vi "test Get All TPDO Communication Parameter.vi"(11 "Test Case In":refnum<class "Test PDO Mapping.lvclass">) -> (0 "error out":errorcluster, 3 "Test Case Out":refnum<class "Test PDO Mapping.lvclass">)   [LabVIEW 2020, in "Test PDO Mapping.lvclass"]
uses:
  Test PDO Mapping.lvclass
  C:/Program Files/National Instruments/LabVIEW 2026/vi.lib/Astemes/LUnit/Test Case.lvclass
  EDS-File-Viewer/source/Electronic Datasheet/Electronic Datasheet.lvclass/Electronic Datasheet.ctl
  <vilib>/Astemes/LUnit/Test Case.lvclass/Test Case.ctl
  source/PDO Communication Parameter/PDO Communication Parameter.lvclass
  4993e8ee-a06a-463a-9684-69129f64d5ce.vi
  EDS-File-Viewer/source/Electronic Datasheet/Electronic Datasheet.lvclass
  source/CANopen.lvlib
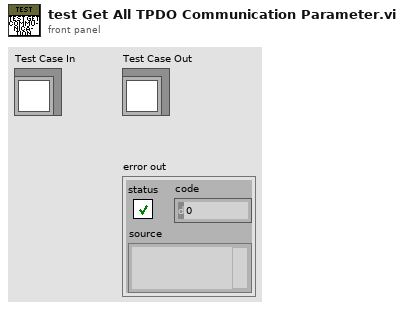
[diagram p1: front panel]
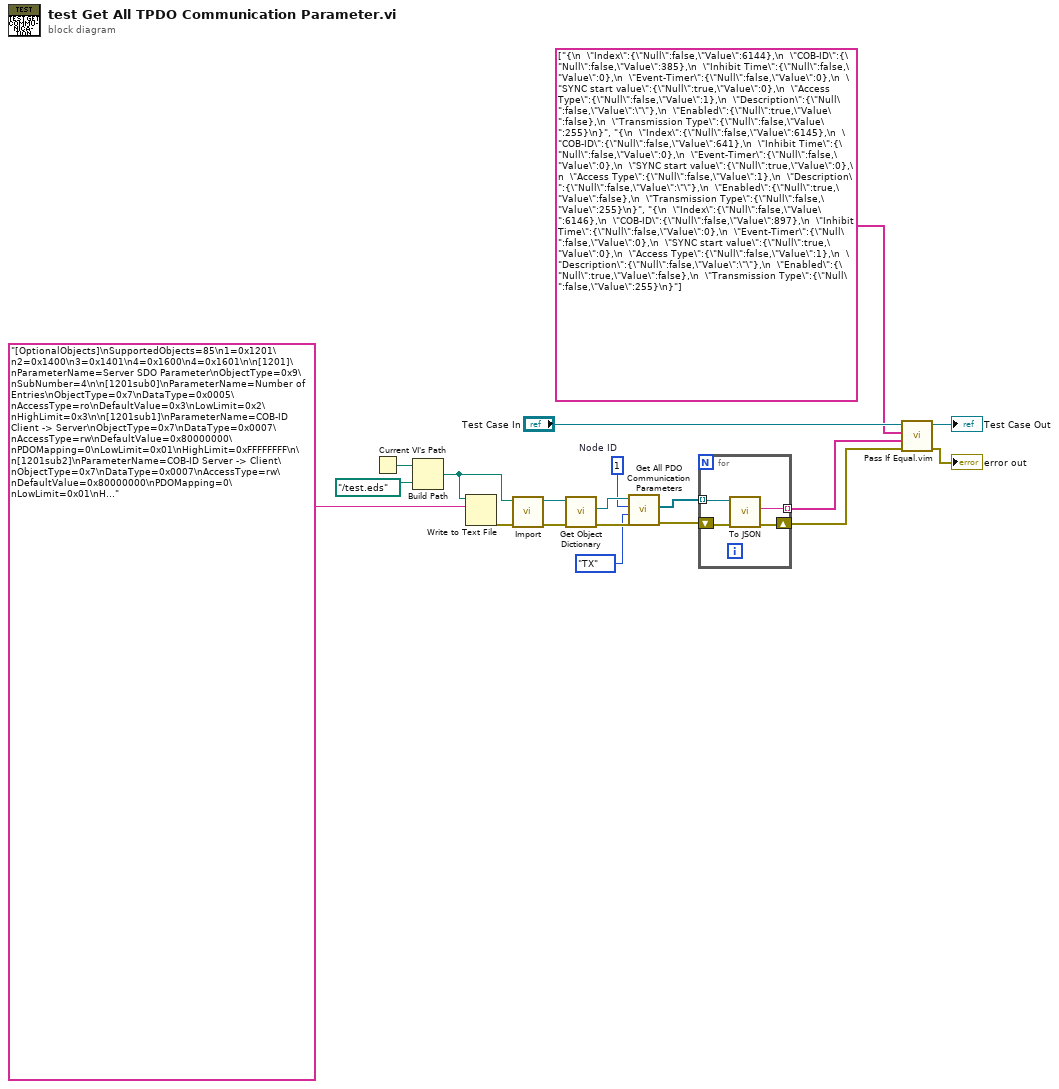
[diagram p0: block diagram]
diagram:
  w7 = u8 1  # Node ID
  n1 = Current VI's Path() -> (path=w16:path)
  n2 = Build Path(base path=w16, name or relative path=path "../test.eds") -> (appended path=w13:path)
  n3 = Write to Text File(file (use dialog)=w13, text="[OptionalObjects]\nSupportedObjects=85\n1=0x1201\n2=0x1400\n3=0x1401\n4=0x1600\n4=0x1601\n\n[1201]\nParameterName=Server SDO Parameter\nObjectType=0x9\nSubNumber=4\n\n[1201sub0]\nParameterName=Number of Entries\nObjectType=0x7\nDataType=0x0005\nAccessType=ro\nDefaultValue=0x3\nLowLimit=0x2\nHighLimit=0x3\n\n[1201sub1]\nParameterName=COB-ID Client -> Server\nObjectType=0x7\nDataType=0x0007\nAccessType=rw\nDefaultValue=0x80000000\nPDOMapping=0\nLowLimit=0x01\nHighLimit=0xFFFFFFFF\n\n[1201sub2]\nParameterName=COB-ID Server -> Client\nObjectType=0x7\nDataType=0x0007\nAccessType=rw\nDefaultValue=0x80000000\nPDOMapping=0\nLowLimit=0x01\nHighLimit=0xFFFFFFFF\n\n[1201sub3]\nParameterName=Node ID of the SDO Client\nObjectType=0x7\nDataType=0x0005\nAccessType=rw\nPDOMapping=0\nLowLimit=1\nHighLimit=127\n\n[1400]\nParameterName=Receive PDO 1 Communication Parameter\nObjectType=0x9\nSubNumber=5\n\n[1400sub0]\nParameterName=Number of Entries\nObjectType=0x7\nDataType=0x0005\nAccessType=ro\nDefaultValue=0x05\nLowLimit=0x02\nHighLimit=0x05\n\n[1400sub1]\nParameterName=COB-ID\nObjectType=0x7\nDataType=0x0007\nAccessType=rw\nDefaultValue=$NODEID+0x00000200\nLowLimit=0x00000001\nHighLimit=0xFFFFFFFF\n\n[1400sub2]\nParameterName=Transmission Type\nObjectType=0x7\nDataType=0x0005\nAccessType=rw\nDefaultValue=0xFF\nLowLimit=0x00\nHighLimit=0xFF\n\n[1400sub3]\nParameterName=Inhibit Time\nObjectType=0x7\nDataType=0x0006\nAccessType=rw\nDefaultValue=0x0000\nLowLimit=0x0000\nHighLimit=0xFFFF\n\n[1400sub5]\nParameterName=Event Timer\nObjectType=0x7\nDataType=0x0006\nAccessType=rw\nDefaultValue=0x0\nLowLimit=0x0\nHighLimit=0xFFFF\n\n[1401]\nParameterName=Receive PDO 2 Communication Parameter\nObjectType=0x9\nSubNumber=5\n\n[1401sub0]\nParameterName=Number of Entries\nObjectType=0x7\nDataType=0x0005\nAccessType=ro\nDefaultValue=0x05\nLowLimit=0x02\nHighLimit=0x05\n\n[1401sub1]\nParameterName=COB-ID\nObjectType=0x7\nDataType=0x0007\nAccessType=rw\nDefaultValue=$NODEID+0x00000300\nLowLimit=0x00000001\nHighLimit=0xFFFFFFFF\n\n[1401sub2]\nParameterName=Transmission Type\nObjectType=0x7\nDataType=0x0005\nAccessType=rw\nDefaultValue=0xFF\nLowLimit=0x00\nHighLimit=0xFF\n\n[1401sub3]\nParameterName=Inhibit Time\nObjectType=0x7\nDataType=0x0006\nAccessType=rw\nDefaultValue=0x0000\nLowLimit=0x0000\nHighLimit=0xFFFF\n\n[1401sub5]\nParameterName=Event Timer\nObjectType=0x7\nDataType=0x0006\nAccessType=rw\nDefaultValue=0x0\nLowLimit=0x0\nHighLimit=0xFFFF\n\n[1600]\nParameterName=Receive PDO 1 Mapping Parameter\nObjectType=0x9\nSubNumber=9\n\n[1600sub0]\nParameterName=Number of Entries\nObjectType=0x7\nDataType=0x0005\nAccessType=rw\nDefaultValue=8\nLowLimit=0\nHighLimit=64\n\n[1600sub1]\nParameterName=PDO Mapping Entry\nObjectType=0x7\nDataType=0x0007\nAccessType=rw\nDefaultValue=0x62000108\nLowLimit=0x00000000\nHighLimit=0xFFFFFFFF\n\n[1600sub2]\nParameterName=PDO Mapping Entry\nObjectType=0x7\nDataType=0x0007\nAccessType=rw\nDefaultValue=0x62000208\nLowLimit=0x00000000\nHighLimit=0xFFFFFFFF\n\n[1600sub3]\nParameterName=PDO Mapping Entry\nObjectType=0x7\nDataType=0x0007\nAccessType=rw\nDefaultValue=0x62000308\nLowLimit=0x00000000\nHighLimit=0xFFFFFFFF\n\n[1600sub4]\nParameterName=PDO Mapping Entry\nObjectType=0x7\nDataType=0x0007\nAccessType=rw\nDefaultValue=0x62000408\nLowLimit=0x00000000\nHighLimit=0xFFFFFFFF\n\n[1600sub5]\nParameterName=PDO Mapping Entry\nObjectType=0x7\nDataType=0x0007\nAccessType=rw\nDefaultValue=0x62000508\nLowLimit=0x00000000\nHighLimit=0xFFFFFFFF\n\n[1600sub6]\nParameterName=PDO Mapping Entry\nObjectType=0x7\nDataType=0x0007\nAccessType=rw\nDefaultValue=0x62000608\nLowLimit=0x00000000\nHighLimit=0xFFFFFFFF\n\n[1600sub7]\nParameterName=PDO Mapping Entry\nObjectType=0x7\nDataType=0x0007\nAccessType=rw\nDefaultValue=0x62000708\nLowLimit=0x00000000\nHighLimit=0xFFFFFFFF\n\n[1600sub8]\nParameterName=PDO Mapping Entry\nObjectType=0x7\nDataType=0x0007\nAccessType=rw\nDefaultValue=0x62000808\nLowLimit=0x00000000\nHighLimit=0xFFFFFFFF\n\n[1601]\nParameterName=Receive PDO 2 Mapping Parameter\nObjectType=0x9\nSubNumber=9\n\n[1601sub0]\nParameterName=Number of Entries\nObjectType=0x7\nDataType=0x0005\nAccessType=rw\nDefaultValue=4\nLowLimit=0\nHighLimit=64\n\n[1601sub1]\nParameterName=PDO Mapping Entry\nObjectType=0x7\nDataType=0x0007\nAccessType=rw\nDefaultValue=0x64110110\nLowLimit=0x00000000\nHighLimit=0xFFFFFFFF\n\n[1601sub2]\nParameterName=PDO Mapping Entry\nObjectType=0x7\nDataType=0x0007\nAccessType=rw\nDefaultValue=0x64110210\nLowLimit=0x00000000\nHighLimit=0xFFFFFFFF\n\n[1601sub3]\nParameterName=PDO Mapping Entry\nObjectType=0x7\nDataType=0x0007\nAccessType=rw\nDefaultValue=0x64110310\nLowLimit=0x00000000\nHighLimit=0xFFFFFFFF\n\n[1601sub4]\nParameterName=PDO Mapping Entry\nObjectType=0x7\nDataType=0x0007\nAccessType=rw\nDefaultValue=0x64110410\nLowLimit=0x00000000\nHighLimit=0xFFFFFFFF\n\n[1601sub5]\nParameterName=PDO Mapping Entry\nObjectType=0x7\nDataType=0x0007\nAccessType=rw\nDefaultValue=0x00000000\nLowLimit=0x00000000\nHighLimit=0xFFFFFFFF\n\n[1601sub6]\nParameterName=PDO Mapping Entry\nObjectType=0x7\nDataType=0x0007\nAccessType=rw\nDefaultValue=0x00000000\nLowLimit=0x00000000\nHighLimit=0xFFFFFFFF\n\n[1601sub7]\nParameterName=PDO Mapping Entry\nObjectType=0x7\nDataType=0x0007\nAccessType=rw\nDefaultValue=0x00000000\nLowLimit=0x00000000\nHighLimit=0xFFFFFFFF\n\n[1601sub8]\nParameterName=PDO Mapping Entry\nObjectType=0x7\nDataType=0x0007\nAccessType=rw\nDefaultValue=0x00000000\nLowLimit=0x00000000\nHighLimit=0xFFFFFFFF\n\n[1800]\nParameterName=Transmit PDO 1 Communication Parameter\nObjectType=0x9\nSubNumber=5\n\n[1800sub0]\nParameterName=Number of Entries\nObjectType=0x7\nDataType=0x0005\nAccessType=ro\nDefaultValue=0x05\nLowLimit=0x02\nHighLimit=0x05\n\n[1800sub1]\nParameterName=COB-ID\nObjectType=0x7\nDataType=0x0007\nAccessType=rw\nDefaultValue=$NODEID+0x00000180\nLowLimit=0x00000001\nHighLimit=0xFFFFFFFF\n\n[1800sub2]\nParameterName=Transmission Type\nObjectType=0x7\nDataType=0x0005\nAccessType=rw\nDefaultValue=0xFF\nLowLimit=0x00\nHighLimit=0xFF\n\n[1800sub3]\nParameterName=Inhibit Time\nObjectType=0x7\nDataType=0x0006\nAccessType=rw\nDefaultValue=0x0000\nLowLimit=0x0000\nHighLimit=0xFFFF\n\n[1800sub5]\nParameterName=Event Timer\nObjectType=0x7\nDataType=0x0006\nAccessType=rw\nDefaultValue=0x0\nLowLimit=0x0\nHighLimit=0xFFFF\n\n[1801]\nParameterName=Transmit PDO 2 Communication Parameter\nObjectType=0x9\nSubNumber=5\n\n[1801sub0]\nParameterName=Number of Entries\nObjectType=0x7\nDataType=0x0005\nAccessType=ro\nDefaultValue=0x05\nLowLimit=0x02\nHighLimit=0x05\n\n[1801sub1]\nParameterName=COB-ID\nObjectType=0x7\nDataType=0x0007\nAccessType=rw\nDefaultValue=$NODEID+0x00000280\nLowLimit=0x00000001\nHighLimit=0xFFFFFFFF\n\n[1801sub2]\nParameterName=Transmission Type\nObjectType=0x7\nDataType=0x0005\nAccessType=rw\nDefaultValue=0xFF\nLowLimit=0x00\nHighLimit=0xFF\n\n[1801sub3]\nParameterName=Inhibit Time\nObjectType=0x7\nDataType=0x0006\nAccessType=rw\nDefaultValue=0x0000\nLowLimit=0x0000\nHighLimit=0xFFFF\n\n[1801sub5]\nParameterName=Event Timer\nObjectType=0x7\nDataType=0x0006\nAccessType=rw\nDefaultValue=0x0\nLowLimit=0x0000\nHighLimit=0xFFFF\n\n[1802]\nParameterName=Transmit PDO 3 Communication Parameter\nObjectType=0x9\nSubNumber=5\n\n[1802sub0]\nParameterName=Number of Entries\nObjectType=0x7\nDataType=0x0005\nAccessType=ro\nDefaultValue=0x05\nLowLimit=0x02\nHighLimit=0x05\n\n[1802sub1]\nParameterName=COB-ID\nObjectType=0x7\nDataType=0x0007\nAccessType=rw\nDefaultValue=$NODEID+0x00000380\nLowLimit=0x00000001\nHighLimit=0xFFFFFFFF\n\n[1802sub2]\nParameterName=Transmission Type\nObjectType=0x7\nDataType=0x0005\nAccessType=rw\nDefaultValue=0xFF\nLowLimit=0x00\nHighLimit=0xFF\n\n[1802sub3]\nParameterName=Inhibit Time\nObjectType=0x7\nDataType=0x0006\nAccessType=rw\nDefaultValue=0x0000\nLowLimit=0x0000\nHighLimit=0xFFFF\n\n[1802sub5]\nParameterName=Event Timer\nObjectType=0x7\nDataType=0x0006\nAccessType=rw\nDefaultValue=0x0\nLowLimit=0x0000\nHighLimit=0xFFFF") -> (error out=w12:errorcluster)  [unwired: 2 in, 2 out]
  n4 = call "Import.vi"("error in"=w12, "EDS File Path"=w13) -> ("error out"=w11:errorcluster, "Electronic Datasheet"=w9:refnum<class "Electronic Datasheet.lvclass">)  [unwired: 8 in]
  n5 = call "Get Object Dictionary.vi"("error in"=w11, "Electronic Datasheet in"=w9) -> ("error out"=w10:errorcluster, "Obj Dict"=w8:refnum<class "Object Dictionary.lvclass">)  [unwired: 7 in, 1 out]
  n6 = call "Get All PDO Communication Parameters.vi"("error in"=w10, "Type"=enum16{"RX", "TX"}."TX", "Node ID"=w7, "Obj Dict in"=w8) -> ("error out"=w4:errorcluster, "PDO Communication Parameters"=w5:refnum<class "PDO Communication Parameter.lvclass">[])  [unwired: 5 in, 1 out]
  n7 = for {
    tunnel: w5 -> [w21] mode=indexing
    shift-right: [w23] -> w3
    shift-left: w4 -> [w22]
    tunnel: [w20] -> w2 mode=indexing
    n8 = call-dynamic "To JSON.vi"("error in"=w22, "PDO Communication Parameter in"=w21) -> ("error out"=w23:errorcluster, "<JSON>"=w20:string)  [unwired: 7 in, 1 out]
  }
  n9 = call "Pass If Equal.vim"("error in (no error)"=w3, "Actual"=w2, "Expected"=string[] ["{\n  \"Index\":{\"Null\":false,\"Value\":6144},\n  \"COB-ID\":{\"Null\":false,\"Value\":385},\n  \"Inhibit Time\":{\"Null\":false,\"Value\":0},\n  \"Event-Timer\":{\"Null\":false,\"Value\":0},\n  \"SYNC start value\":{\"Null\":true,\"Value\":0},\n  \"Access Type\":{\"Null\":false,\"Value\":1},\n  \"Description\":{\"Null\":false,\"Value\":\"\"},\n  \"Enabled\":{\"Null\":true,\"Value\":false},\n  \"Transmission Type\":{\"Null\":false,\"Value\":255}\n}", "{\n  \"Index\":{\"Null\":false,\"Value\":6145},\n  \"COB-ID\":{\"Null\":false,\"Value\":641},\n  \"Inhibit Time\":{\"Null\":false,\"Value\":0},\n  \"Event-Timer\":{\"Null\":false,\"Value\":0},\n  \"SYNC start value\":{\"Null\":true,\"Value\":0},\n  \"Access Type\":{\"Null\":false,\"Value\":1},\n  \"Description\":{\"Null\":false,\"Value\":\"\"},\n  \"Enabled\":{\"Null\":true,\"Value\":false},\n  \"Transmission Type\":{\"Null\":false,\"Value\":255}\n}", "{\n  \"Index\":{\"Null\":false,\"Value\":6146},\n  \"COB-ID\":{\"Null\":false,\"Value\":897},\n  \"Inhibit Time\":{\"Null\":false,\"Value\":0},\n  \"Event-Timer\":{\"Null\":false,\"Value\":0},\n  \"SYNC start value\":{\"Null\":true,\"Value\":0},\n  \"Access Type\":{\"Null\":false,\"Value\":1},\n  \"Description\":{\"Null\":false,\"Value\":\"\"},\n  \"Enabled\":{\"Null\":true,\"Value\":false},\n  \"Transmission Type\":{\"Null\":false,\"Value\":255}\n}"] ("Array"), "LUnit Test Case In"="Test Case In") -> ("error out"=→"error out":errorcluster, "LUnit Test Case Out"=→"Test Case Out":refnum<class "Test PDO Mapping.lvclass">)  [unwired: 6 in]
